vi "Entry.vi"(8 "error in (no error)":errorcluster, 11 "New State":refnum<class "GTH-Holding.lvclass">) -> (0 "error out":errorcluster, 3 "State out":refnum<class "GTH-Holding.lvclass">)   [LabVIEW 2014, in "Elevator.lvlib" / "EL-Go To Height.lvlib" / "GTH-Holding.lvclass"]
doc: "This is an abstract method. Override this method to define the behavior when you enter the state."
uses:
  GTH-Holding.lvclass
  <vilib>/ActorFramework/Actor/Actor.lvclass/Actor.ctl
  <vilib>/ActorFramework/Message Enqueuer/Message Enqueuer.lvclass/Message Enqueuer.ctl
  Elevator Messages/Set Rate (Percent) Msg/Set Rate (Percent) Msg.lvclass/Set Rate (Percent) Msg.ctl
  <vilib>/ActorFramework/Message Enqueuer/Init from Existing Queue.vi
  <vilib>/ActorFramework/Message Enqueuer/Enqueue.vi
  <vilib>/ActorFramework/Message Priority Queue/Priority Enqueue.vi
  EL-Go To Height Class/EL-Go To Height.lvclass
  <vilib>/ActorFramework/Message Enqueuer/Message Enqueuer.lvclass
  Elevator Messages/Set Rate (Percent) Msg/Set Rate (Percent) Msg.lvclass
  Robot Actor Framework/Command Actor/Command Actor Messages/FInished Command Msg/Finish Command Msg.lvclass
  <vilib>/ActorFramework/Actor/Actor.lvclass
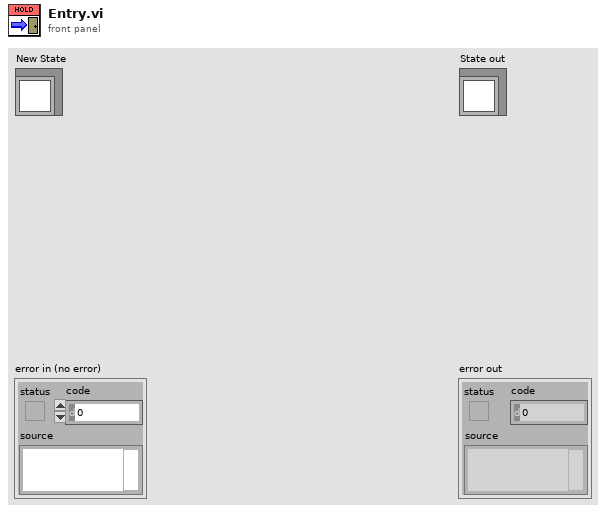
[diagram p1: front panel]
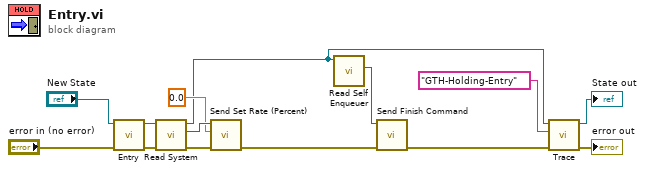
[diagram p0: block diagram]
diagram:
  n1 = call-parent "Entry.vi"("error in (no error)"="error in (no error)", "New State"="New State") -> ("error out"=w6:errorcluster, "State out"=w9:refnum<class "GTH-Holding.lvclass">)  [unwired: 8 in]
  n2 = call-dynamic "Read System.vi"("error in (no error)"=w6, "Command in"=w9) -> ("error out"=w5:errorcluster, "Actor Framework:Message Enqueuer"=w8:refnum<class "Message Enqueuer.lvclass">, "Command out"=w4:refnum<class "GTH-Holding.lvclass">)  [unwired: 7 in]
  n3 = call "Send Set Rate (Percent).vi"("error in (no error)"=w5, "Percent"=0.0, "Message Enqueuer"=w8) -> ("error out"=w2:errorcluster)  [unwired: 7 in, 1 out]
  n4 = call <vilib>:"Read Self Enqueuer.vi"("Actor"=w4) -> ("Self Enqueuer"=w3:refnum<class "Message Enqueuer.lvclass">)  [unwired: 10 in]
  n5 = call "Send Finish Command.vi"("error in (no error)"=w2, "Message Enqueuer"=w3) -> ("error out"=w1:errorcluster)  [unwired: 8 in, 1 out]
  n6 = call-dynamic "Trace.vi"("error in (no error)"=w1, "Command Action"="GTH-Holding-Entry", "Command Actor in"=w4) -> ("error out"=→"error out":errorcluster, "Command Actor out"=→"State out":refnum<class "GTH-Holding.lvclass">)  [unwired: 7 in]
